vi "macro_DiffDrivePoseEst2_Execute.vi"() -> ()   [LabVIEW 2019, in "Trajectory_Library.lvlib"]
uses:
  Trajectory_Library.lvlib
  TypeDef/TRANSLATION2D.ctl
  TypeDef/ROTATION2D.ctl
  TypeDef/POSE2D.ctl
panel:
  in  "Vision TImeStamp_Seconds":dbl=0.02
  in  "visionRobotPose":T1={"TRANSLATION"={"X"=0.0, "Y"=0.0}, "ROTATION"={"VALUE"=0.0, "COS"=1.0, "SIN"=0.0}} {"ROTATION"."SIN" format="%13.4f"; "ROTATION"."COS" format="%13.4f"; "ROTATION"."VALUE" format="%13.4f"; "TRANSLATION"."Y" format="%14.3f"; "TRANSLATION"."X" format="%14.3f"}
  in  "Add Vision Meas":bool
  in  "Game Started":bool=TRUE
  in  "InitialPose":T1={"TRANSLATION"={"X"=0.0, "Y"=0.0}, "ROTATION"={"VALUE"=0.0, "COS"=1.0, "SIN"=0.0}} {"ROTATION"."SIN" format="%13.4f"; "ROTATION"."COS" format="%13.4f"; "ROTATION"."VALUE" format="%13.4f"; "TRANSLATION"."Y" format="%14.3f"; "TRANSLATION"."X" format="%14.3f"}
  in  "Gyro Degrees":dbl
  in  "RightDistance_M":dbl=0.02
  in  "LeftDistance_M":dbl=0.02
  out "Estimated Pose":T1={"TRANSLATION"={"X"=0.0, "Y"=0.0}, "ROTATION"={"VALUE"=0.0, "COS"=1.0, "SIN"=0.0}} {"ROTATION"."SIN" format="%13.4f"; "ROTATION"."COS" format="%13.4f"; "ROTATION"."VALUE" format="%13.4f"; "TRANSLATION"."Y" format="%14.3f"; "TRANSLATION"."X" format="%14.3f"}
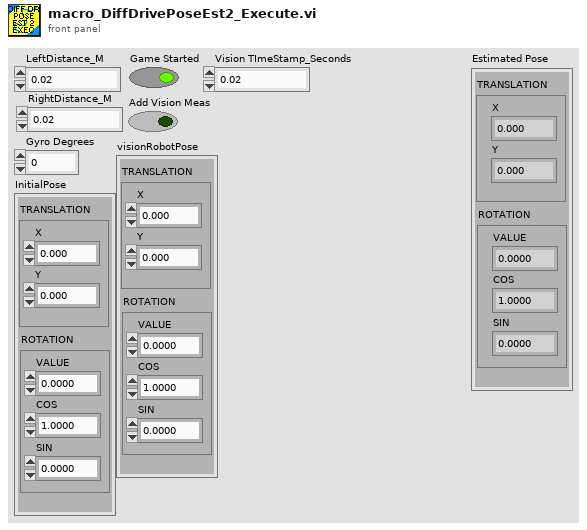
[diagram p1: front panel]
types:
  T1 = typedef "Trajectory_Library.lvlib/POSE2D.ctl" = cluster{"TRANSLATION":T2, "ROTATION":T3}
  T2 = typedef "Trajectory_Library.lvlib/TRANSLATION2D.ctl" = cluster{"X":dbl, "Y":dbl}
  T3 = typedef "Trajectory_Library.lvlib/ROTATION2D.ctl" = cluster{"VALUE":dbl, "COS":dbl, "SIN":dbl}
  T4 = typedef "Trajectory_Library.lvlib/DIFF_DRIVE_POSE_EST2_CONFIG.ctl" = cluster{"TrackWidth_Meters":dbl, "Odom X std dev M":dbl, "Odom Y std dev M":dbl, "Odom Heading std dev Rad":dbl, "Vision X std dev M":dbl, "Vision Y std dev M":dbl, "Vision Heading std dev Rad":dbl}
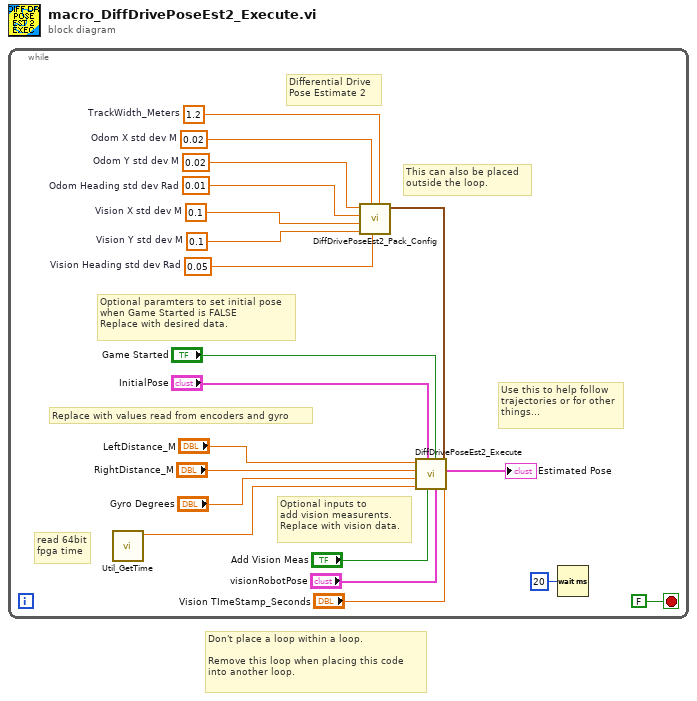
[diagram p0: block diagram]
diagram:
  # "Don't place a loop within a loop.\n \nRemove this loop when placing this code\ninto another loop."
  n1 = while {
    stop <- FALSE stop-if-true
    w11 = 0.02  # Odom Y std dev M
    w12 = 0.01  # Odom Heading std dev Rad
    w13 = 0.1  # Vision X std dev M
    w14 = 0.1  # Vision Y std dev M
    w15 = 0.02  # Odom X std dev M
    w16 = 0.05  # Vision Heading std dev Rad
    w17 = 1.2  # TrackWidth_Meters
    # "Optional inputs to\nadd vision measurents.\nReplace with vision data."
    # "Replace with values read from encoders and gyro"
    # "Optional paramters to set initial pose\nwhen Game Started is FALSE\nReplace with desired data."
    # "read 64bit\nfpga time"
    # "This can also be placed \noutside the loop."
    # "Use this to help follow\ntrajectories or for other\nthings..."
    # "Differential Drive \nPose Estimate 2"
    n2 = call "Util_GetTime.vi"() -> ("FPGA_Time_Seconds"=w6:dbl)  [unwired: 9 in, 2 out]
    n3 = call "DiffDrivePoseEst2_Pack_Config.vi"("TrackWidth_Meters"=w17, "Vision Heading std dev Rad"=w16, "Odom X std dev M"=w15, "Vision Y std dev M"=w14, "Vision X std dev M"=w13, "Odom Heading std dev Rad"=w12, "Odom Y std dev M"=w11) -> ("DiffPoseEst2Config"=w18:T4)  [unwired: 4 in]
    n4 = call "DiffDrivePoseEst2_Execute.vi"("Vision TImeStamp_Seconds"="Vision TImeStamp_Seconds", "DiffPoseEst2Config"=w18, "visionRobotPose"="visionRobotPose", "Game Started"="Game Started", "Add Vision Meas"="Add Vision Meas", "InitialPose"="InitialPose", "Pass Through Time"=w6, "Gyro Degrees"="Gyro Degrees", "RightDistance_M"="RightDistance_M", "LeftDistance_M"="LeftDistance_M") -> ("Estimated Pose"=→"Estimated Pose":T1)  [unwired: 1 out]
    n5 = Wait (ms)(milliseconds to wait=u32 20) -> ()  [unwired: 1 out]
  }
